vi "Analyze.vi"(8 "error in (no error)":errorcluster, 10 "Image in":T1, 11 "Analyze SHG-AK in":refnum<class "Analyze SHG-AK.lvclass">) -> (0 "error out":errorcluster, 1 "Result":refnum<class "Analyze Results Base.lvclass">, 2 "Image out":T1, 3 "Analyze SHG-AK out":refnum<class "Analyze SHG-AK.lvclass">)   [LabVIEW 2014, in "Analyze.lvlib" / "Analyze SHG-AK.lvclass"]
uses:
  Analyze SHG-AK.lvclass
  <vilib>/vision/Image Controls.llb/IMAQ Image.ctl
  Results and Overlays/Results Base/Analyze Results Base.lvclass
  Results and Overlays/Results SHG-AK/Analyze Results SHG-AK.lvclass
  Results and Overlays/Results Base/Analyze Results Base.lvclass/Analyze Results Base.ctl
  Results and Overlays/Results SHG-AK/Analyze Results SHG-AK.lvclass/Analyze Results SHG-AK.ctl
  Results and Overlays/Results Base/Write Position.vi
  Results and Overlays/Results SHG-AK/Write Gaussian Fit.vi
  Results and Overlays/Results SHG-AK/Write FWHM .vi
  Results and Overlays/Results SHG-AK/Write X-Values.vi
  Results and Overlays/Results SHG-AK/Write FWHM Gaussfit.vi
  Results and Overlays/Results SHG-AK/Write Y-ROI Averages.vi
  Analyze BaseClass/Analyze BaseClass/Analyze BaseClass.lvclass
  <vilib>/vision/NI_Vision_Development_Module.lvlib
  <vilib>/Analysis/NI_AALPro.lvlib
  Utility/POLARIS Vision utility.lvlib
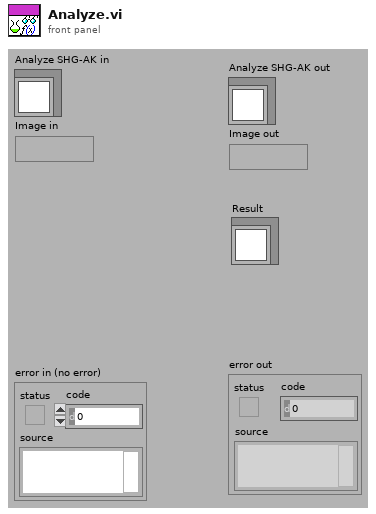
[diagram p1: front panel]
types:
  T1 = typedef "IMAQ Image.ctl" = refnum<image>
  T2 = typedef "ROI Descriptor" = cluster{"Global Rectangle":i32[], "Contours":cluster{"ID":enum32{"External", "Internal"}, "Type":u32, "Coordinates":i32[]}[]}
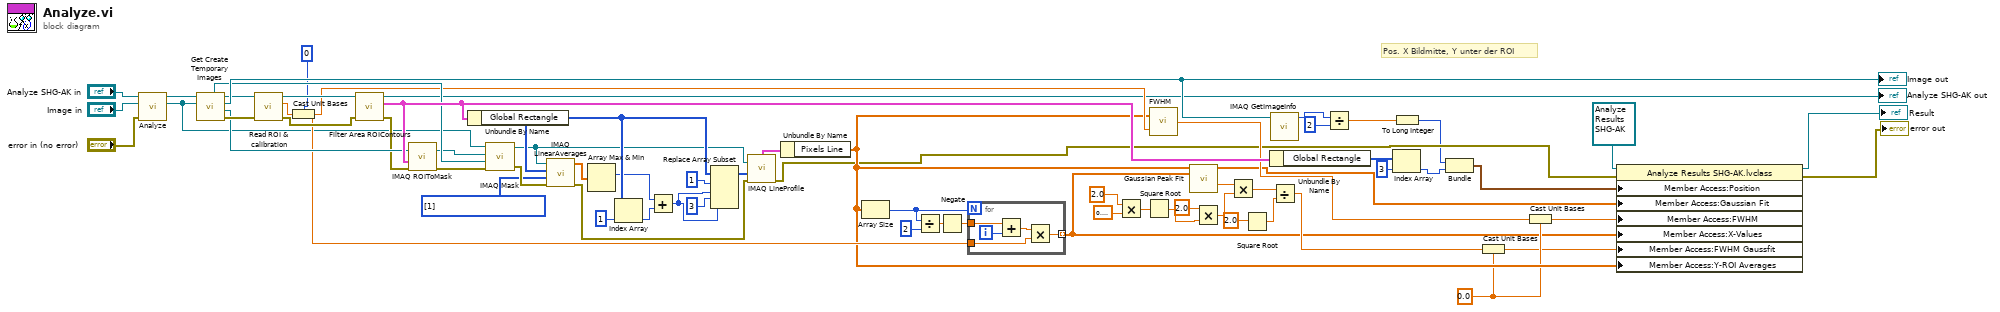
[diagram p0: block diagram]
diagram:
  w7 = dbl[unit] 0.0 ("unit (none)")
  w42 = i32[] [1] items=["X Axis Averages", "Y Axis Averages", "X + Y Axis Averages", "X - Y Axis Averages"] ("Averages")
  # "Pos. X Bildmitte, Y unter der ROI"
  n1 = call-parent "Analyze.vi"("error in (no error)"="error in (no error)", "Image in"="Image in", "Analyze BaseClass in"="Analyze SHG-AK in") -> ("Image out"=w22:T1, "Analyze BaseClass out"=w23:refnum<class "Analyze SHG-AK.lvclass">)  [unwired: 5 in, 2 out]
  n2 = call-dynamic "Get Create Temporary Images.vi"("Image in"=w22, "Analyze BaseClass in"=w23) -> ("error out"=w51:errorcluster, "image mask"=w50:T1, "work image"=w54:T1, "Analyze BaseClass out"=w52:refnum<class "Analyze SHG-AK.lvclass">, "masked image"=w49:T1)  [unwired: 5 in]
  "Image out" <- w54
  n3 = call-dynamic "Read ROI & calibration.vi"("error in (no error)"=w51, "Analyze BaseClass in"=w52) -> ("error out"=w45:errorcluster, "calibration mm/px"=w28:dbl[unit], "Analyze BaseClass out"=w46:refnum<class "Analyze SHG-AK.lvclass">)  [unwired: 6 in, 1 out]
  n4 = Cast Unit Bases(0:w28, 1:0) -> (2:w29:dbl)
  n5 = call-dynamic "Filter Area ROIContours.vi"("error in (no error)"=w45, "Analyze BaseClass in"=w46) -> ("error out"=w44:errorcluster, "ROI of Area type"=w53:T2, "Analyze BaseClass out"=→"Analyze SHG-AK out":refnum<class "Analyze SHG-AK.lvclass">)  [unwired: 7 in]
  n6 = call "IMAQ ROIToMask"("error in (no error)"=w44, "ROI Descriptor"=w53, "Image"=w50) -> ("error out"=w48:errorcluster, "Image Out"=w47:T1)  [unwired: 3 in, 1 out]
  n7 = Unbundle By Name(w53) -> ("Global Rectangle"=w38:i32[])
  n8 = call "IMAQ Mask"("error in (no error)"=w48, "Image Dst"=w49, "Image Mask"=w47, "Image Src"=w22) -> ("error out"=w43:errorcluster, "Image Dst Out"=w33:T1)  [unwired: 1 in]
  n9 = call "IMAQ LinearAverages"("error in (no error)"=w43, "Averages"=w42, "Optional Rectangle"=w38, "Image Src"=w33) -> ("error out"=w31:errorcluster, "Y Axis Averages"=w41:sgl[])  [unwired: 3 in, 3 out]
  n10 = Array Max & Min(array=w41) -> (max index (indices)=w35:i32)  [unwired: 3 out]
  n11 = Index Array(array=w38, index=1) -> (element=w36:i32)
  n12 = Add(x=w35, y=w36) -> (x+y=w34:i32)
  n13 = Replace Array Subset(array=w38, new element #1=w34, index #1=1 ("index"), new element #2=w34, index #2=3 ("index")) -> (w32:i32[])
  n14 = call "IMAQ LineProfile"("error in (no error)"=w31, "Line Coordinates"=w32, "Image"=w33) -> ("error out"=w17:errorcluster, "Line Graph"=w30:cluster{"x0":sgl, "dx":sgl, "Pixels Line":sgl[]})  [unwired: 2 in, 2 out]
  n15 = Unbundle By Name(w30) -> ("Pixels Line"=w18:sgl[])
  n16 = Array Size(array=w18) -> (size(s)=w56:i32)
  n17 = Divide(x=w56, y=2) -> (x/y=w58:dbl)
  n18 = Negate(x=w58) -> (-x=w55:dbl)
  n19 = for {
    N: w56 -> [_]
    tunnel: w55 -> [w72]
    tunnel: [w70] -> w5 mode=indexing
    tunnel: w29 -> [w69]
    i -> [w73]
    n20 = Add(x=w72, y=w73) -> (x+y=w71:dbl)
    n21 = Multiply(x=w71, y=w69) -> (x*y=w70:dbl)
  }
  n22 = Multiply(x=2.0 ("y"), y=0.6931471805599453) -> (x*y=w61:dbl)
  n23 = Square Root(x=w61) -> (sqrt(x)=w62:dbl)
  n24 = call "FWHM.vi"("calibration"=w29, "array"=w18) -> ("FHWM"=w20:dbl)
  n25 = call <vilib>:"Gaussian Peak Fit.vi"("Y"=w18, "X"=w5) -> ("Best Gaussian Fit"=w9:dbl[], "standard deviation"=w68:dbl)  [unwired: 7 in, 5 out]
  n26 = Multiply(x=2.0 ("y"), y=w62) -> (x*y=w63:dbl)
  n27 = Multiply(x=w68, y=w63) -> (x*y=w66:dbl)
  n28 = Square Root(x=2.0) -> (sqrt(x)=w65:dbl)
  n29 = Unbundle By Name(w53) -> ("Global Rectangle"=w16:i32[])
  n30 = call "IMAQ GetImageInfo"("Image"=w54) -> ("X Resolution"=w15:i32)  [unwired: 3 in, 7 out]
  n31 = Divide(x=w66, y=w65) -> (x/y=w19:dbl)
  n32 = Divide(x=w15, y=2) -> (x/y=w13:dbl)
  n33 = To Long Integer(number=w13) -> (32bit integer=w10:i32)
  n34 = Index Array(array=w16, index=3) -> (element=w12:i32)
  n35 = Bundle(w10, w12) -> (w8:cluster{i32, i32})  [unwired: 1 in]
  n36 = Cast Unit Bases(0:w19, 1:w7) -> (2:w6:dbl[unit])
  n37 = Cast Unit Bases(0:w20, 1:w7) -> (2:w4:dbl[unit])
  n38 = property class="Analyze Results SHG-AK.lvclass"(reference=refnum<class "Analyze Results SHG-AK.lvclass"> refnum ("Analyze Results SHG-AK.lvclass"), error in=w17, "Member Access:Position"=w8, "Member Access:Gaussian Fit"=w9, "Member Access:FWHM "=w4, "Member Access:X-Values"=w5, "Member Access:FWHM Gaussfit"=w6, "Member Access:Y-ROI Averages"=w18) -> (reference out=→"Result":refnum<class "Analyze Results SHG-AK.lvclass">, error out=→"error out":errorcluster)
